vi "fix sync item names.vi"(11 "sync items in":T1[](array[typedef])) -> (3 "sync items out":T1[](array[typedef]))   [LabVIEW 2013, in "Shared Memory editor node.lvclass"]
uses:
  Shared Memory editor node.lvclass
  sync/sync item.ctl
  sync/sync mechanism.ctl
  module/configuration/Shared Memory configuration.lvclass
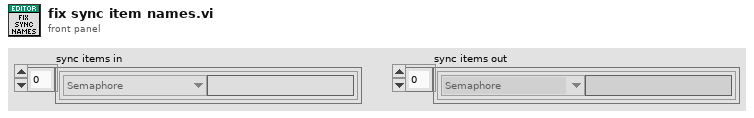
[diagram p1: front panel]
types:
  T1 = typedef "Shared Memory configuration.lvclass/sync item.ctl" = cluster{"mechanism":T2, "name":string}
  T2 = typedef "Shared Memory configuration.lvclass/sync mechanism.ctl" = enum16{"Semaphore"}
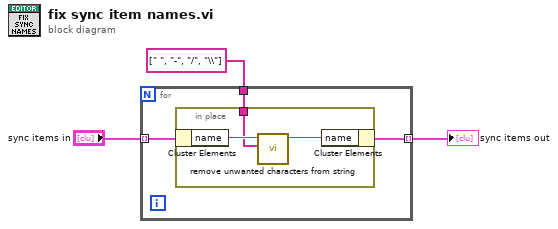
[diagram p0: block diagram]
diagram:
  n1 = for {
    tunnel: "sync items in" -> [w6] mode=indexing
    tunnel: string[] [" ", "-", "/", "\\"] ("unwanted patterns/characters") -> [w5]
    tunnel: [w4] -> w3 mode=indexing
    n2 = in-place {
      in-place-border: w5 -> [w7]
      n3 = in-place-cluster #1(w6) -> ("name"=w9:string)
      n4 = call "remove unwanted characters from string.vi"("unwanted patterns/characters"=w7, "string in"=w9) -> ("string out"=w8:string)  [unwired: 9 in]
      n5 = in-place-cluster #1("name"=w8) -> (w4:T1)
    }
  }
  "sync items out" <- w3
